vi "ClustersAndVectors.vi"() -> ()   [LabVIEW 2014]
panel:
  out "XY Graph":cluster{i32, i32}[](graph)
  in  "Domínio":i32
  out "Array":i32[](array[numeric])
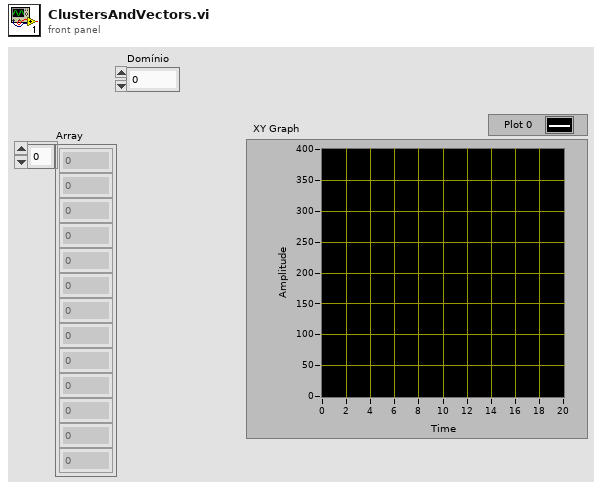
[diagram p1: front panel]
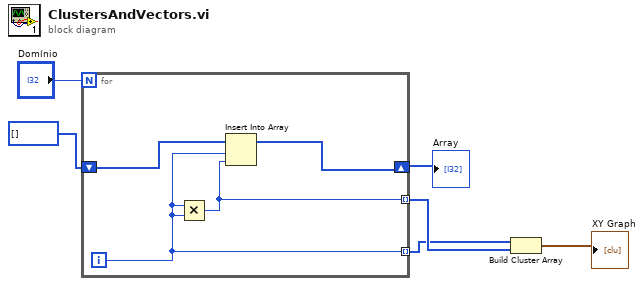
[diagram p0: block diagram]
diagram:
  n1 = for {
    N: "Domínio" -> [_]
    shift-right: [w10] -> w6
    shift-left: i32[] [] -> [w9]
    tunnel: [w8] -> w2 mode=indexing
    tunnel: [w7] -> w1 mode=indexing
    i -> [w7]
    n2 = Multiply(x=w7, y=w7) -> (x*y=w8:i32)
    n3 = Insert Into Array(array=w9, index=w7, new element=w8) -> (w10:i32[])
  }
  "Array" <- w6
  n4 = Build Cluster Array(w1, w2) -> (→"XY Graph":cluster{i32, i32}[])
